vi "add_Wrench.vi"(4 "Wrench":T1, 5 "msg in":string) -> (2 "msg out":string)   [LabVIEW 2015]
doc: "Flattens a wrench into a message"
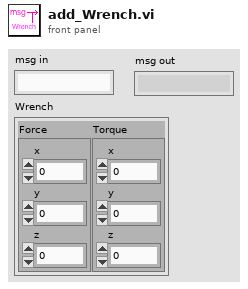
[diagram p1: front panel]
types:
  T1 = cluster{"Force":cluster{"x":dbl, "y":dbl, "z":dbl}, "Torque":cluster{"x":dbl, "y":dbl, "z":dbl}}
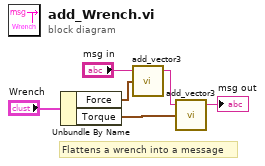
[diagram p0: block diagram]
diagram:
  # "Flattens a wrench into a message"
  n1 = Unbundle By Name("Wrench") -> ("Force"=w2:cluster{"x":dbl, "y":dbl, "z":dbl}, "Torque"=w1:cluster{"x":dbl, "y":dbl, "z":dbl})
  n2 = call "add_vector3.vi"("Vector3"=w2, "msg in"="msg in") -> ("msg out"=w5:string)  [unwired: 3 in]
  n3 = call "add_vector3.vi"("Vector3"=w1, "msg in"=w5) -> ("msg out"=→"msg out":string)  [unwired: 3 in]
